vi "Calibrate1.vi"   [LabVIEW 2019]
uses:
  <vilib>/Utility/file.llb/Write Delimited Spreadsheet (I64).vi
  Robot Global Data.vi
types:
  T1 = typedef "WPI_AnalogChannelDevRef.ctl" = cluster{"DevStatus":errorcluster, "Analog Channel":T2}
  T2 = typedef "FPGA_AIChannel.ctl" = enum8{"AI 0", "AI 1", "AI 2", "AI 3", "AI MXP 0", "AI MXP 1", "AI MXP 2", "AI MXP 3", "Invalid"}
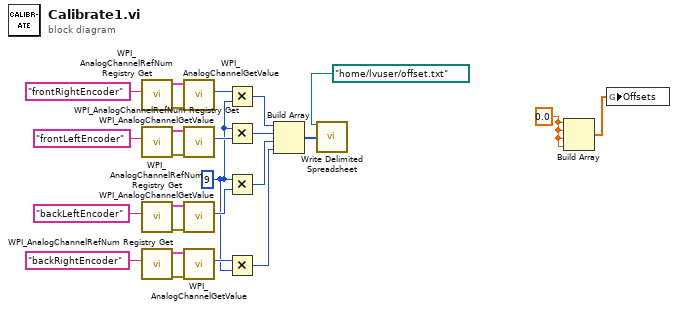
[diagram p0: block diagram]
diagram:
  w2 = 0.0
  w3 = i16 9 ("y")
  n1 = call <vilib>:"WPI_AnalogChannelRefNum Registry Get.vi"("refnum name"="frontRightEncoder") -> ("error out"=w17:errorcluster, "AIDeviceRef"=w18:T1)  [unwired: 9 in]
  n2 = call <vilib>:"WPI_AnalogChannelRefNum Registry Get.vi"("refnum name"="frontLeftEncoder") -> ("error out"=w23:errorcluster, "AIDeviceRef"=w24:T1)  [unwired: 9 in]
  n3 = call <vilib>:"WPI_AnalogChannelRefNum Registry Get.vi"("refnum name"="backLeftEncoder") -> ("error out"=w15:errorcluster, "AIDeviceRef"=w16:T1)  [unwired: 9 in]
  n4 = call <vilib>:"WPI_AnalogChannelRefNum Registry Get.vi"("refnum name"="backRightEncoder") -> ("error out"=w13:errorcluster, "AIDeviceRef"=w14:T1)  [unwired: 9 in]
  n5 = call <vilib>:"WPI_AnalogChannelGetValue.vi"("error in (no error)"=w17, "AIDeviceRef"=w18) -> ("Value"=w11:i16)  [unwired: 7 in, 2 out]
  n6 = call <vilib>:"WPI_AnalogChannelGetValue.vi"("error in (no error)"=w23, "AIDeviceRef"=w24) -> ("Value"=w10:i16)  [unwired: 7 in, 2 out]
  n7 = call <vilib>:"WPI_AnalogChannelGetValue.vi"("error in (no error)"=w15, "AIDeviceRef"=w16) -> ("Value"=w9:i16)  [unwired: 7 in, 2 out]
  n8 = call <vilib>:"WPI_AnalogChannelGetValue.vi"("error in (no error)"=w13, "AIDeviceRef"=w14) -> ("Value"=w8:i16)  [unwired: 7 in, 2 out]
  n9 = Multiply(x=w11, y=w3) -> (x*y=w7:i16)
  n10 = Multiply(x=w3, y=w10) -> (x*y=w6:i16)
  n11 = Multiply(x=w3, y=w9) -> (x*y=w5:i16)
  n12 = Multiply(x=w8, y=w3) -> (x*y=w4:i16)
  n13 = Build Array(w7, w6, w5, w4) -> (w12:i16[])
  n14 = call-poly <vilib>:"Write Delimited Spreadsheet.vi"("file path (dialog if empty)"=path "/home/lvuser/offset.txt", "1D data"=w12) -> ()  [unwired: 12 in, 2 out]
  n15 = Build Array(w2, w2, w2, w2) -> (w1:dbl[])
  n16 = global write "Robot Global Data.vi" "Offsets"(w1) -> ()
